vi "Radians to Ticks.vi"(1 "Radians":dbl) -> (0 "Ticks":dbl)   [LabVIEW 2016]
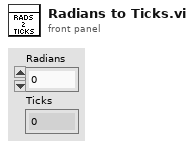
[diagram p1: front panel]
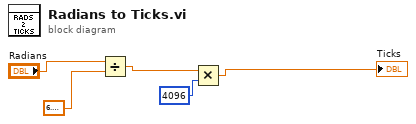
[diagram p0: block diagram]
diagram:
  n1 = Divide(x="Radians", y=6.283185307179586) -> (x/y=w2:dbl)
  n2 = Multiply(x=w2, y=4096) -> (x*y=→"Ticks":dbl)
